vi "GetFileFlowProcess.vi"(8 "error in (no error)":errorcluster, 11 "source":string) -> (0 "error out":errorcluster, 1 "found":bool, 2 "last block":bool, 3 "Fileflow process":string)   [LabVIEW 2017, in "FileFlow.lvlib"]
uses:
  <vilib>/addons/InsightCM/Devices/Shared/Common/FileFlow/FileFlow.lvlib
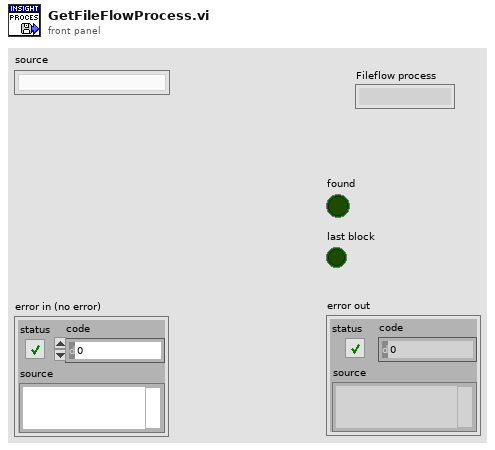
[diagram p1: front panel]
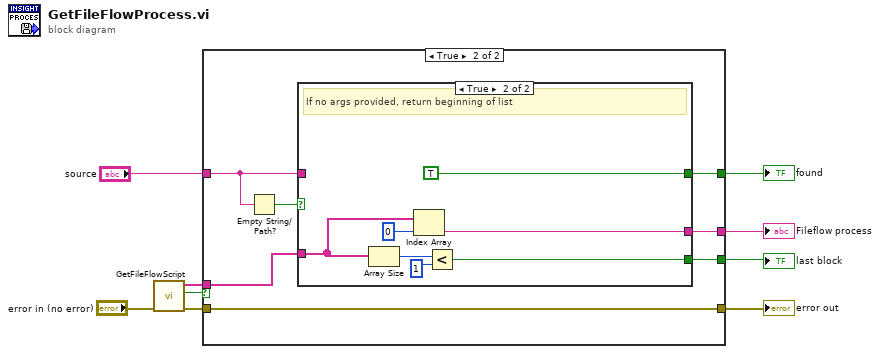
[diagram p0: block diagram]
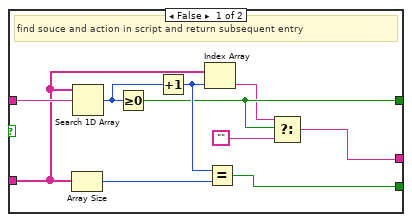
[diagram p3: hidden frame]
diagram:
  n1 = call <vilib>:"GetFileFlowScript.vi"("error in (no error)"="error in (no error)") -> ("error out"=w3:errorcluster, "found"=w2:bool, "Fileflow script"=w1:string[])  [unwired: 8 in]
  n2 = case shown="True" w2 {
    selector: w2 -> [w11 _]
    tunnel: [w10 w13] -> w9
    tunnel: [w11 w17] -> w8
    tunnel: w3 -> [w10 w13]
    tunnel: "source" -> [_ w15]
    tunnel: [_ w18] -> w6
    tunnel: [_ w16] -> w5
    tunnel: w1 -> [_ w12]
    frame False {
    }
    frame True {
      n3 = Empty String/Path?(string/path=w15) -> (empty?=w14:bool)
      n4 = case shown="True" w14 {
        tunnel: w15 -> [w28 _]
        tunnel: [w19 w34] -> w18
        tunnel: [w22 TRUE] -> w17
        tunnel: w12 -> [w25 w33]
        tunnel: [w27 w30] -> w16
        frame False {
          # "find souce and action in script and return subsequent entry"
          n5 = Array Size(array=w25) -> (size(s)=w24:i32)
          n6 = Search 1D Array(1D array=w25, element=w28) -> (index of element=w26:i32)  [unwired: 1 in]
          n7 = Greater Or Equal To 0?(x=w26) -> (x >= 0?=w22:bool)
          n8 = Increment(x=w26) -> (x+1=w23:i32)
          n9 = Index Array(array=w25, index=w23) -> (element=w20:string)
          n10 = Equal?(x=w23, y=w24) -> (x = y?=w27:bool)
          n11 = Select(t=w20, s=w22, f="") -> (s? t:f=w19:string)
        }
        frame True {
          # "If no args provided, return beginning of list"
          n12 = Array Size(array=w33) -> (size(s)=w32:i32)
          n13 = Index Array(array=w33, index=0) -> (element=w34:string)
          n14 = Less?(x=w32, y=1) -> (x < y?=w30:bool)
        }
      }
    }
  }
  "error out" <- w9
  "found" <- w8
  "Fileflow process" <- w6
  "last block" <- w5
